vi "CMD_LOADTOOL.vi"(6 "Gantry in":refnum<class "Gantry.lvclass">, 8 "error in (no error)":errorcluster, 10 "Arguments":string[](array[string]), 11 "gScript Interpreter in":refnum<class "gScript Interpreter.lvclass">) -> (0 "error out":errorcluster, 3 "gScript Interpreter out":refnum<class "gScript Interpreter.lvclass">, 4 "Gantry out":refnum<class "Gantry.lvclass">)   [LabVIEW 2017, in "gScript Interpreter.lvclass"]
uses:
  gScript Interpreter.lvclass
  Shared Components/Gantry Class/Gantry.lvclass
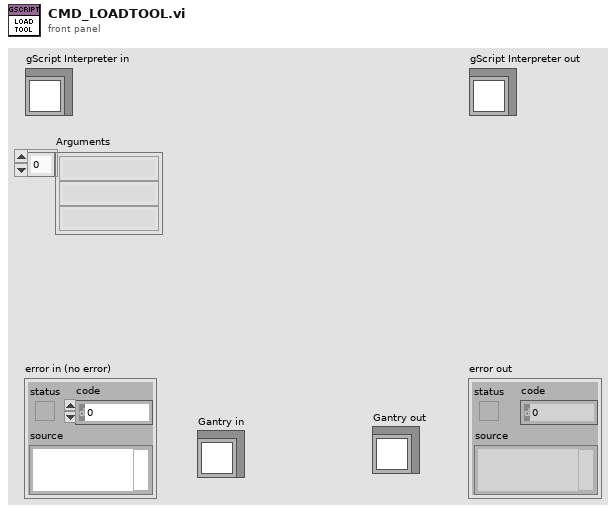
[diagram p1: front panel]
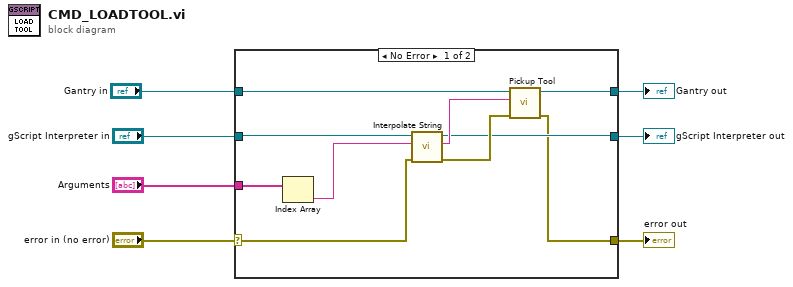
[diagram p0: block diagram]
diagram:
  n1 = case shown="No Error" "error in (no error)" {
    selector: "error in (no error)" -> [w12 w20]
    tunnel: [w8 w20] -> w6
    tunnel: [w9 w19] -> w4
    tunnel: "gScript Interpreter in" -> [w14 w19]
    tunnel: "Arguments" -> [w17 _]
    tunnel: "Gantry in" -> [w16 w18]
    tunnel: [w15 w18] -> w1
    frame No Error {
      n2 = Index Array(array=w17) -> (element=w13:string)  [unwired: 1 in]
      n3 = call-dynamic "Interpolate String.vi"("error in (no error)"=w12, "Input String"=w13, "gScript Interpreter in"=w14) -> ("error out"=w11:errorcluster, "Output String"=w10:string, "gScript Interpreter out"=w9:refnum<class "gScript Interpreter.lvclass">)  [unwired: 6 in]
      n4 = call-dynamic "Pickup Tool.vi"("error in"=w11, "Tool"=w10, "Gantry in"=w16) -> ("error out"=w8:errorcluster, "Gantry out"=w15:refnum<class "Gantry.lvclass">)  [unwired: 7 in]
    }
    frame Error {
    }
  }
  "error out" <- w6
  "gScript Interpreter out" <- w4
  "Gantry out" <- w1
